vi "Command Execution Response.vi"(8 "error in":errorcluster, 10 "Reply Payload":T1) -> (0 "error out":errorcluster)   [LabVIEW 2015, in "LV-WinSCP.lvlib"]
doc: "This broadcast is fired when the specified command finished executing on the distant target.\nIt returns the command status information and error messages if any.\nSent command and standard output are also returned.\n\n_____\nCreated using DQMH Event Scripter 6.1.0.128."
uses:
  LV-WinSCP.lvlib
  Execute Command On Target (Reply Payload)--cluster.ctl
  Classes/CommandExecution/Status.ctl
  Classes/CommandExecution/ErrorDescription.ctl
  Classes/CommandExecution/Command Execution.lvclass
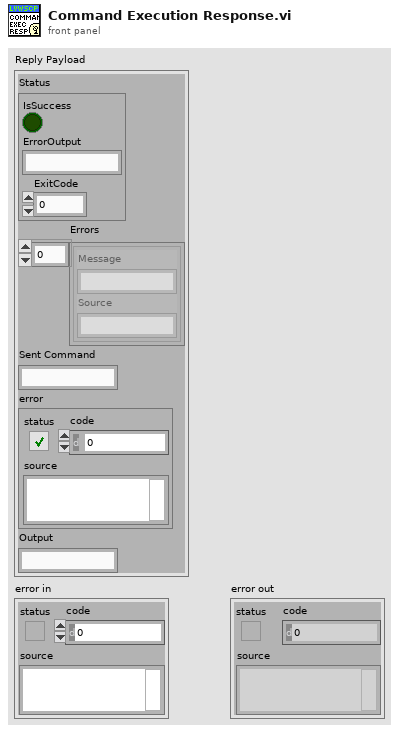
[diagram p1: front panel]
types:
  T1 = typedef "LV-WinSCP.lvlib/Execute Command On Target (Reply Payload)--cluster.ctl" = cluster{"Status":T2, "Errors":T3[], "Sent Command":string, "error":errorcluster, "Output":string}
  T2 = typedef "WinSCP.lvlib/Command Execution.lvclass/Status.ctl" = cluster{"IsSuccess":bool, "ErrorOutput":string, "ExitCode":i32}
  T3 = typedef "WinSCP.lvlib/Command Execution.lvclass/ErrorDescription.ctl" = cluster{"Message":string, "Source":string}
  T4 = typedef "LV-WinSCP.lvlib/Broadcast Events--cluster.ctl" = cluster{"Module Did Init":refnum<user-event>, "Status Updated":refnum<user-event>, "Error Reported":refnum<user-event>, "Module Did Stop":refnum<user-event>, "Update Module Execution Status":refnum<user-event>, "Transfer From Target Status":refnum<user-event>, "Command Execution Response":refnum<user-event>, "Transfer To Target Status":refnum<user-event>}
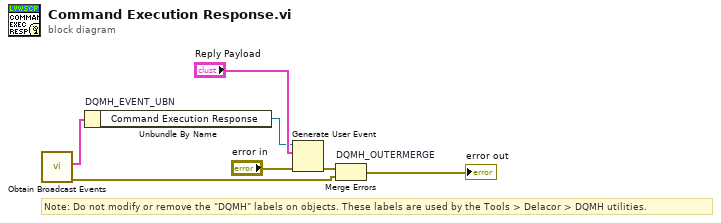
[diagram p0: block diagram]
diagram:
  # "Note: Do not modify or remove the \"DQMH\" labels on objects. These labels are used by the Tools > Delacor > DQMH utilities."
  n1 = call "Obtain Broadcast Events.vi"() -> ("error out"=w2:errorcluster, "LV-WinSCP Broadcast Events"=w1:T4)  [unwired: 10 in]
  n2 = Unbundle By Name "DQMH_EVENT_UBN"(w1) -> ("Command Execution Response"=w4:refnum<user-event>)
  n3 = Generate User Event(user event=w4, event data cluster="Reply Payload", error in="error in") -> (error out=w3:errorcluster)  [unwired: 1 in, 1 out]
  n4 = Merge Errors "DQMH_OUTERMERGE"(w3, w2) -> (→"error out":errorcluster)
